vi "Set Outgoing Work Dispatcher.vi"(8 "error in (no error)":errorcluster, 10 "Work Dispatcher":refnum<class "Work Dispatcher.lvclass">, 11 "Worker In":refnum<class "Worker.lvclass">) -> (0 "error out":errorcluster, 3 "Worker Out":refnum<class "Worker.lvclass">)   [LabVIEW 2020, in "Worker.lvclass"]
uses:
  Worker.lvclass
  C:/Program Files (x86)/National Instruments/LabVIEW 2020/vi.lib/Asteme/Triarc Framework/Process/Process.lvclass
  Work Dispatcher/Work Dispatcher.lvclass
  <vilib>/Asteme/Triarc Framework/Process/Process.lvclass/Process.ctl
  <vilib>/Asteme/Triarc Framework/Process/Public/Lifecycle/Get Lifecycle State.vi
  <vilib>/Utility/error.llb/Clear Errors.vi
  <vilib>/Utility/error.llb/Error Cluster From Error Code.vi
  <vilib>/Asteme/Triarc Framework/Process/Process.lvclass
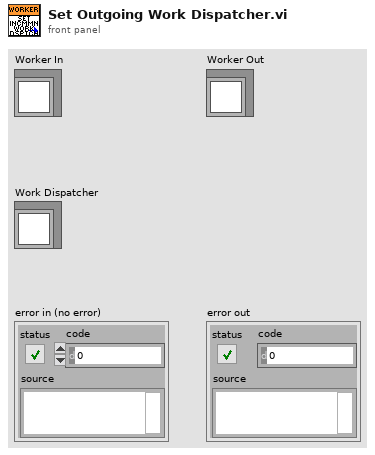
[diagram p1: front panel]
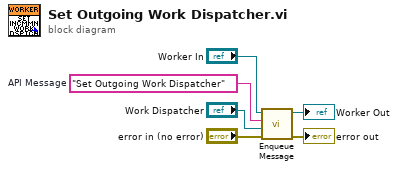
[diagram p0: block diagram]
diagram:
  w3 = "Set Outgoing Work Dispatcher"  # API Message
  n1 = call <vilib>:"Enqueue Message.vi"("error in (no error)"="error in (no error)", "Message Data"="Work Dispatcher", "Message"=w3, "Process In"="Worker In") -> ("error out"=→"error out":errorcluster, "Process Out"=→"Worker Out":refnum<class "Worker.lvclass">)  [unwired: 6 in]
